vi "Find Panel VI Ref.vi"(8 "error in (no error)":errorcluster, 11 "Panel in":refnum<class "Panel.lvclass">) -> (0 "error out":errorcluster, 2 "Panel VI":refnum<vi>, 3 "Panel out":refnum<class "Panel.lvclass">)   [LabVIEW 2020, in "OOPanel.lvlib" / "Panel.lvclass"]
uses:
  Panel.lvclass
  <vilib>/Utility/error.llb/Error Cluster From Error Code.vi
  <vilib>/ErrorRing/Error Ring.xnode
  <vilib>/Utility/Data Type/NI_Data Type.lvlib
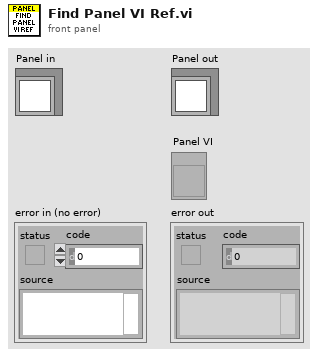
[diagram p1: front panel]
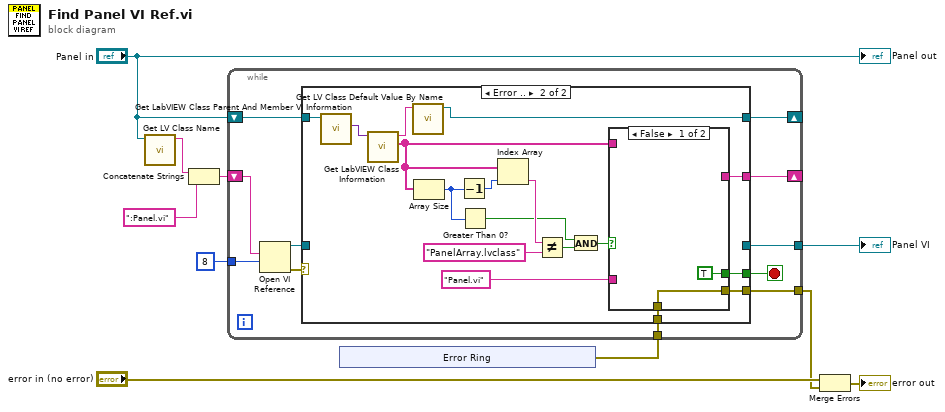
[diagram p0: block diagram]
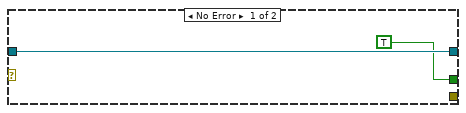
[diagram p2: hidden frame]
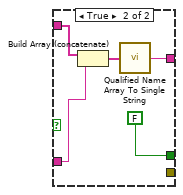
[diagram p3: hidden frame]
diagram:
  n1 = call <vilib>:"Get LV Class Name.vi"("object"="Panel in") -> ("class name"=w9:string)  [unwired: 9 in, 1 out]
  n2 = Concatenate Strings(w9, ":Panel.vi" ("string")) -> (w7:string)
  n3 = xnode "Error Ring"() -> ("error out"=w4:errorcluster)
  n4 = while {
    shift-right: [w15] -> _
    shift-left: w7 -> [w21]
    tunnel: [w18] -> w6
    shift-right: [w11] -> _
    shift-left: "Panel in" -> [w17]
    tunnel: 8 ("options") -> [w16]
    tunnel: w4 -> [w13]
    tunnel: [w12] -> w2
    stop <- w14 stop-if-true
    n5 = Open VI Reference(vi path=w21, options=w16) -> (vi reference=w19:refnum<vi>, error out=w20:errorcluster)  [unwired: 4 in]
    n6 = case shown="Error .." w20 {
      tunnel: w19 -> [w23 _]
      tunnel: [w23 _] -> w18
      tunnel: w17 -> [_ w40]
      tunnel: [_ w32] -> w15
      tunnel: [TRUE w31] -> w14
      tunnel: w13 -> [_ w30]
      tunnel: [_ w29] -> w12
      tunnel: [_ w27] -> w11
      frame No Error {
      }
      frame Error {
        n7 = call <vilib>:"Get LabVIEW Class Parent And Member VI Information.vi"("variant"=w40) -> ("parent class"=w39:variant)  [unwired: 8 in, 2 out]
        n8 = call <vilib>:"Get LabVIEW Class Information.vi"("variant"=w39) -> ("qualified LabVIEW class name"=w33:string[], "LabVIEW class file name"=w28:string)  [unwired: 8 in, 1 out]
        n9 = call <vilib>:"Get LV Class Default Value By Name.vi"("class name"=w28) -> ("object"=w27:refnum<class>)  [unwired: 9 in, 1 out]
        n10 = Array Size(array=w33) -> (size(s)=w26:i32)
        n11 = Decrement(x=w26) -> (x-1=w38:i32)
        n12 = Greater Than 0?(x=w26) -> (x > 0?=w24:bool)
        n13 = Index Array(array=w33, index=w38) -> (element=w37:string)
        n14 = Not Equal?(x=w37, y="PanelArray.lvclass") -> (x != y?=w35:bool)
        n15 = And(x=w24, y=w35) -> (x .and. y?=w25:bool)
        n16 = case shown="False" w25 {
          tunnel: "Panel.vi" -> [_ w46]
          tunnel: w33 -> [_ w47]
          tunnel: [_ w44] -> w32
          tunnel: [TRUE FALSE] -> w31
          tunnel: w30 -> [w41 _]
          tunnel: [w41 _] -> w29
          frame False {
          }
          frame True {
            n17 = Build Array (concatenate)(w47, w46) -> (w45:string[])
            n18 = call <vilib>:"Qualified Name Array To Single String.vi"("Fully Qualified Array"=w45) -> ("Fully Qualified String"=w44:string)
          }
        }
      }
    }
  }
  "Panel VI" <- w6
  n19 = Merge Errors("error in (no error)", w2) -> (→"error out":errorcluster)
  "Panel out" <- "Panel in"
